vi "Single_Omit.vi"(3 "Accept In":bool[](array[boolean]), 4 "Data Values":string[](array[string]), 5 "Omit Strings":string[](array[string])) -> (0 "Accept Out":bool[](array[boolean]))   [LabVIEW 2014]
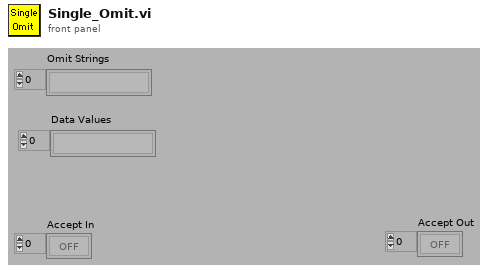
[diagram p1: front panel]
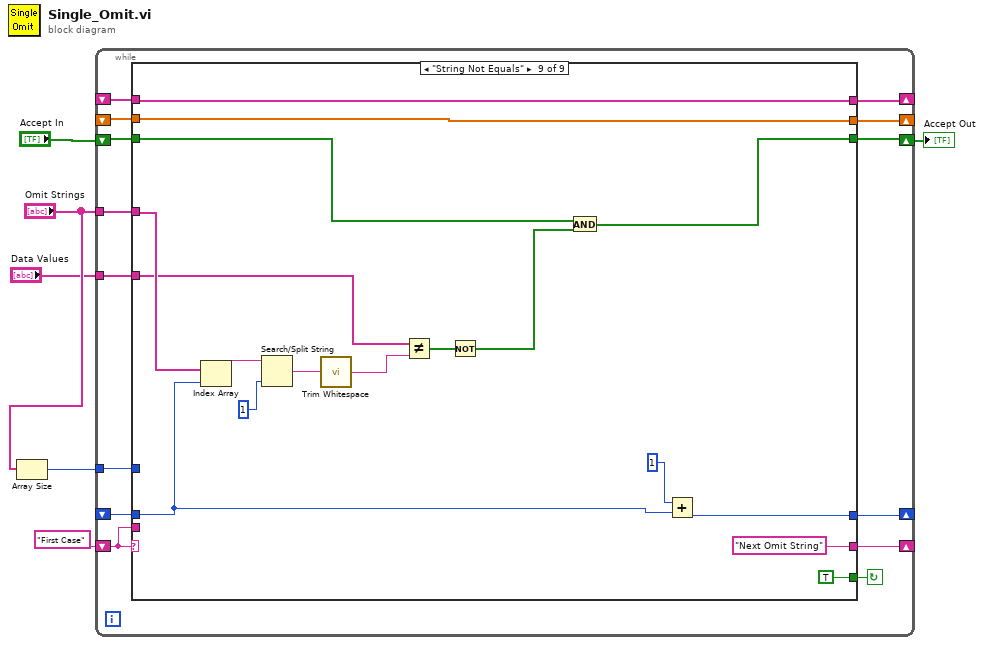
[diagram p0: block diagram]
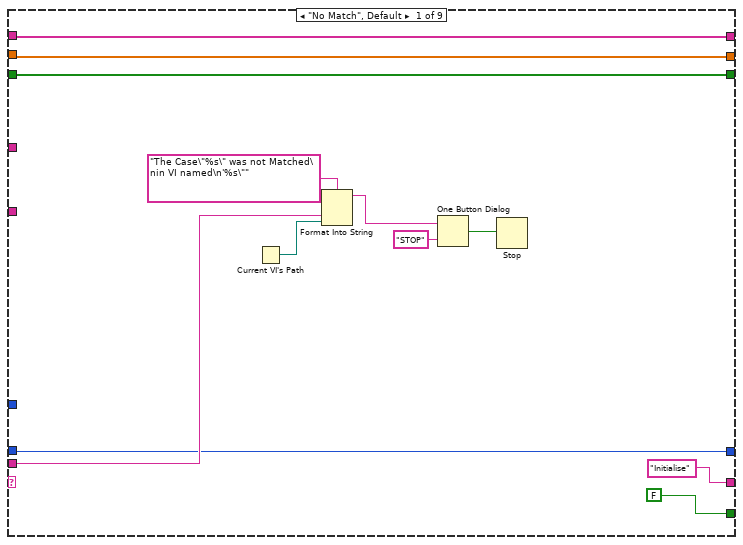
[diagram p2: hidden frame]
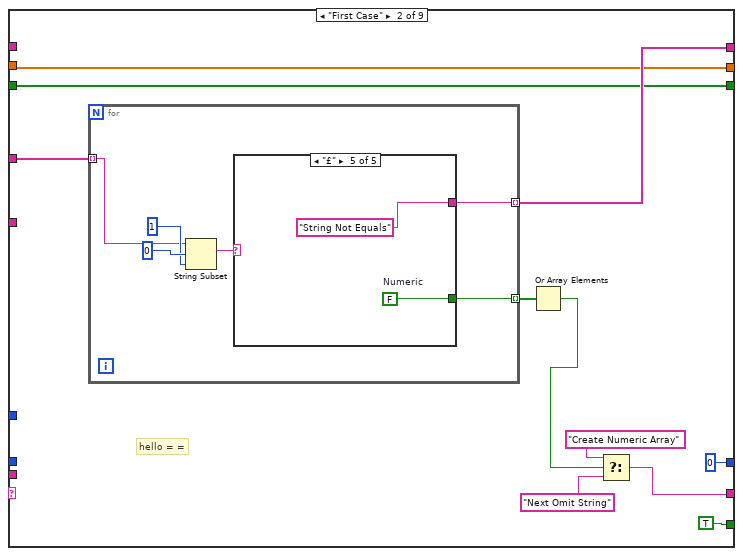
[diagram p3: hidden frame]
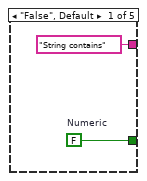
[diagram p4: hidden frame]
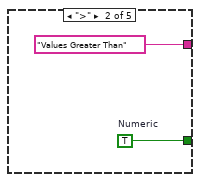
[diagram p5: hidden frame]
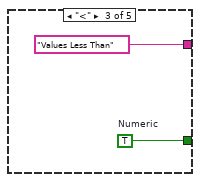
[diagram p6: hidden frame]
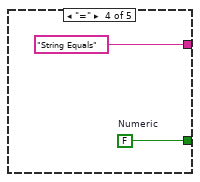
[diagram p7: hidden frame]
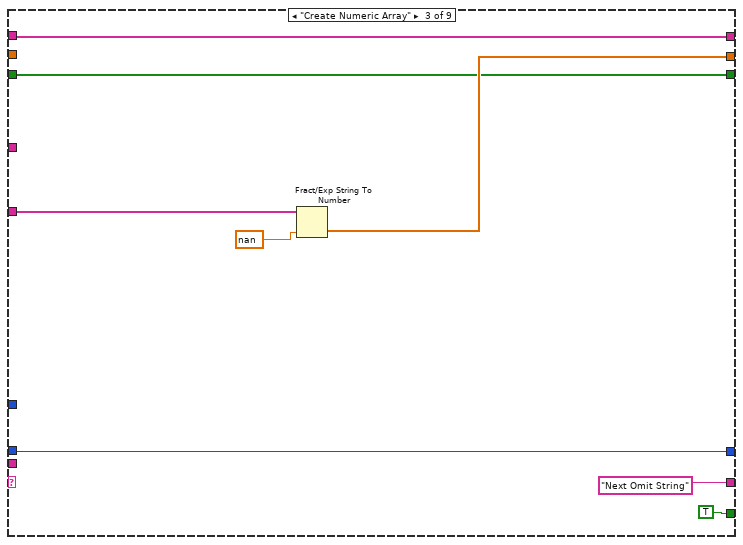
[diagram p8: hidden frame]
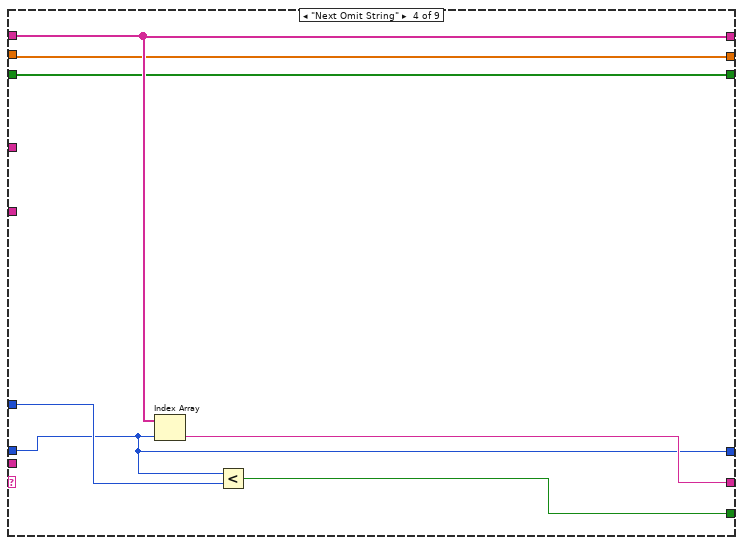
[diagram p9: hidden frame]
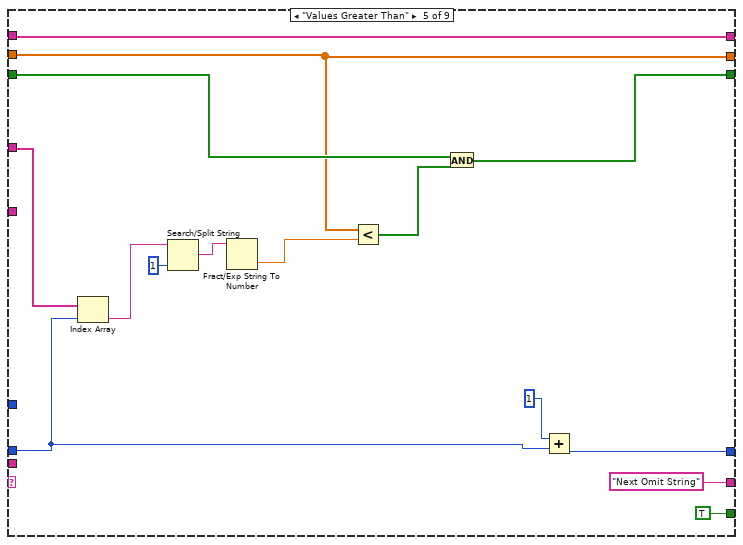
[diagram p10: hidden frame]
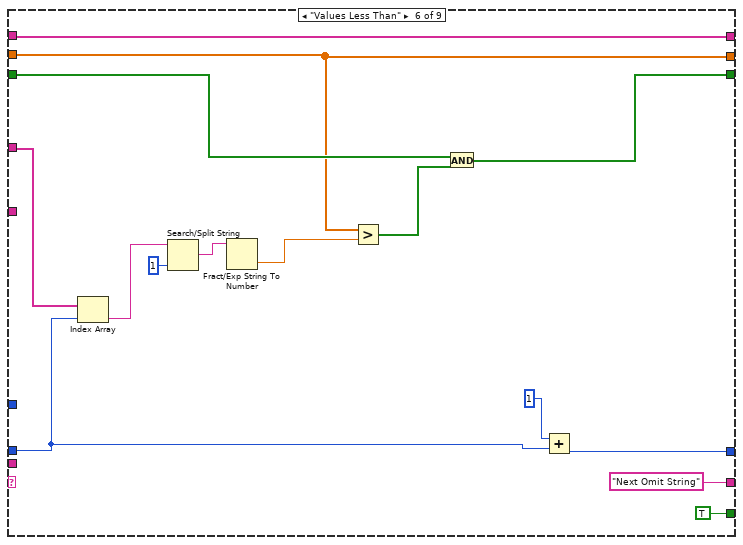
[diagram p11: hidden frame]
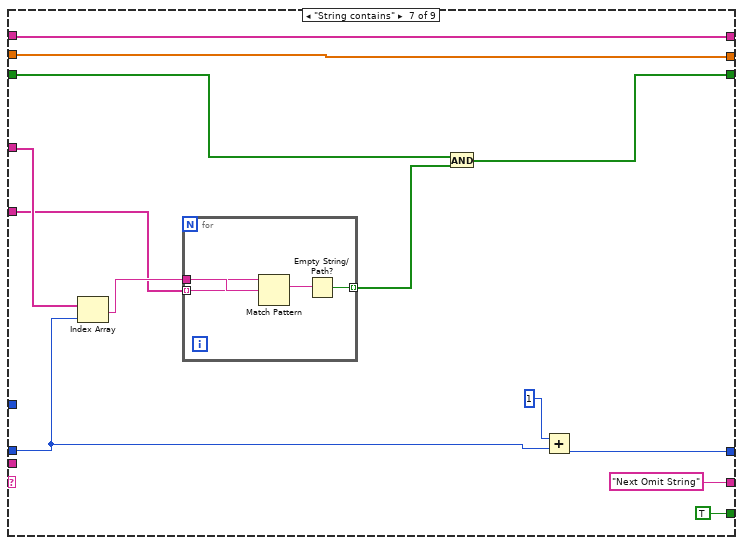
[diagram p12: hidden frame]
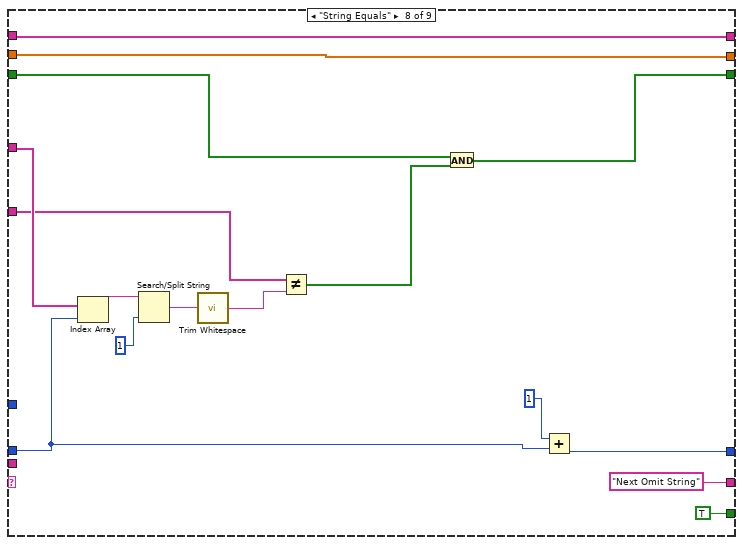
[diagram p13: hidden frame]
diagram:
  n1 = Array Size(array="Omit Strings") -> (size(s)=w3:i32)
  n2 = while {
    shift-left: "Accept In" -> [w7]
    shift-right: [w8] -> w2
    tunnel: w3 -> [w10]
    shift-left: _ -> [w9]
    shift-right: [w11] -> _
    tunnel: "Data Values" -> [w12]
    shift-left: _ -> [w13]
    shift-right: [w14] -> _
    tunnel: "Omit Strings" -> [w15]
    shift-left: _ -> [w17]
    shift-right: [w16] -> _
    shift-left: "First Case" -> [w18]
    shift-right: [w19] -> _
    stop <- w20 continue-if-true
    n3 = case shown="\"String Not Equals\"" w18 {
      tunnel: [FALSE TRUE TRUE w73 TRUE TRUE TRUE TRUE TRUE] -> w20
      tunnel: ["Initialise" w36 "Next Omit String" w72 "Next Omit String" "Next Omit String" "Next Omit String" "Next Omit String" "Next Omit String"] -> w19
      tunnel: w18 -> [w27 _ _ _ _ _ _ _ _]
      tunnel: w17 -> [w24 _ w62 w70 w80 w95 w114 w134 w151]
      tunnel: [w24 w37 w62 w70 w80 w95 w114 w134 w151] -> w16
      tunnel: w15 -> [_ w42 _ _ w88 w103 w117 w137 w154]
      tunnel: [w21 0 w64 w71 w77 w92 w111 w131 w148] -> w14
      tunnel: w13 -> [w21 _ w64 w71 w79 w94 w113 w133 w150]
      tunnel: w12 -> [_ _ w66 _ _ _ w106 w123 w140]
      tunnel: [w23 w35 w65 w69 w81 w96 w108 w128 w145] -> w11
      tunnel: w10 -> [_ _ _ w74 _ _ _ _ _]
      tunnel: w9 -> [w23 w35 _ w69 w81 w96 w108 w128 w145]
      tunnel: [w22 w33 w61 w68 w82 w97 w115 w135 w152] -> w8
      tunnel: w7 -> [w22 w33 w61 w68 w83 w98 w116 w136 w153]
      frame "No Match", Default {
        n4 = Current VI's Path() -> (path=w26:path)
        n5 = Format Into String(format string="The Case\"%s\" was not Matched\nin VI named\n'%s\"" ("Format String"), w27, w26) -> (resulting string=w30:string)  [unwired: 2 in, 1 out]
        n6 = One Button Dialog(message=w30, button name ("OK")="STOP") -> (true=w28:bool)
        n7 = Stop(stop? (T)=w28) -> ()
      }
      frame "First Case" {
        # "hello = ="
        n8 = for {
          tunnel: w42 -> [w46] mode=indexing
          tunnel: [w45] -> w37 mode=indexing
          tunnel: [w44] -> w41 mode=indexing
          n9 = String Subset(string=w46, offset (0)=0, length (rest)=1 ("length")) -> (substring=w47:string)
          n10 = case shown="\"£\"" w47 {
            tunnel: ["String contains" "Values Greater Than" "Values Less Than" "String Equals" "String Not Equals"] -> w45
            tunnel: [w50 w52 w54 w56 w58] -> w44
            frame "False", Default {
              w50 = FALSE  # Numeric
            }
            frame ">" {
              w52 = TRUE  # Numeric
            }
            frame "<" {
              w54 = TRUE  # Numeric
            }
            frame "=" {
              w56 = FALSE  # Numeric
            }
            frame "£" {
              w58 = FALSE  # Numeric
            }
          }
        }
        n11 = Or Array Elements(Boolean array=w41) -> (logical OR=w40:bool)
        n12 = Select(t="Create Numeric Array", s=w40, f="Next Omit String") -> (s? t:f=w36:string)
      }
      frame "Create Numeric Array" {
        n13 = Fract/Exp String To Number(string=w66, default (0 dbl)=nan) -> (number=w65:dbl[])  [unwired: 3 out]
      }
      frame "Next Omit String" {
        n14 = Index Array(array=w70, index=w71) -> (element=w72:string)
        n15 = Less?(x=w71, y=w74) -> (x < y?=w73:bool)
      }
      frame "Values Greater Than" {
        n16 = Index Array(array=w88, index=w79) -> (element=w87:string)
        n17 = Search/Split String(string=w87, offset (0)=1) -> (match + rest of string=w86:string)  [unwired: 3 out]
        n18 = Fract/Exp String To Number(string=w86) -> (number=w85:dbl)  [unwired: 4 out]
        n19 = Less?(x=w81, y=w85) -> (x < y?=w84:bool[])
        n20 = And(x=w83, y=w84) -> (x .and. y?=w82:bool[])
        n21 = Add(x=1, y=w79) -> (x+y=w77:i32)
      }
      frame "Values Less Than" {
        n22 = Index Array(array=w103, index=w94) -> (element=w102:string)
        n23 = Search/Split String(string=w102, offset (0)=1) -> (match + rest of string=w101:string)  [unwired: 3 out]
        n24 = Fract/Exp String To Number(string=w101) -> (number=w100:dbl)  [unwired: 4 out]
        n25 = Greater?(x=w96, y=w100) -> (0:w99:bool[])
        n26 = And(x=w98, y=w99) -> (x .and. y?=w97:bool[])
        n27 = Add(x=1, y=w94) -> (x+y=w92:i32)
      }
      frame "String contains" {
        n28 = Index Array(array=w117, index=w113) -> (element=w107:string)
        n29 = for {
          tunnel: w107 -> [w121]
          tunnel: w106 -> [w120] mode=indexing
          tunnel: [w118] -> w105 mode=indexing
          n30 = Match Pattern(string=w120, regular expression=w121) -> (match substring=w119:string)  [unwired: 4 out]
          n31 = Empty String/Path?(string/path=w119) -> (empty?=w118:bool)
        }
        n32 = And(x=w116, y=w105) -> (x .and. y?=w115:bool[])
        n33 = Add(x=1, y=w113) -> (x+y=w111:i32)
      }
      frame "String Equals" {
        n34 = Index Array(array=w137, index=w133) -> (element=w126:string)
        n35 = Search/Split String(string=w126, offset (0)=1) -> (match + rest of string=w125:string)  [unwired: 3 out]
        n36 = call <vilib>:"Trim Whitespace.vi"("string"=w125) -> ("trimmed string"=w124:string)  [unwired: 1 in]
        n37 = Not Equal?(x=w123, y=w124) -> (x != y?=w122:bool[])
        n38 = And(x=w136, y=w122) -> (x .and. y?=w135:bool[])
        n39 = Add(x=1, y=w133) -> (x+y=w131:i32)
      }
      frame "String Not Equals" {
        n40 = Index Array(array=w154, index=w150) -> (element=w143:string)
        n41 = Search/Split String(string=w143, offset (0)=1) -> (match + rest of string=w142:string)  [unwired: 3 out]
        n42 = call <vilib>:"Trim Whitespace.vi"("string"=w142) -> ("trimmed string"=w141:string)  [unwired: 1 in]
        n43 = Not Equal?(x=w140, y=w141) -> (x != y?=w139:bool[])
        n44 = Not(x=w139) -> (.not. x?=w138:bool[])
        n45 = And(x=w153, y=w138) -> (x .and. y?=w152:bool[])
        n46 = Add(x=1, y=w150) -> (x+y=w148:i32)
      }
    }
  }
  "Accept Out" <- w2
